vi "TimeManager.vi"(10 "Reset?":bool) -> (1 "Start Time":u32, 3 "Time Since Reset":u32)   [LabVIEW 2014]
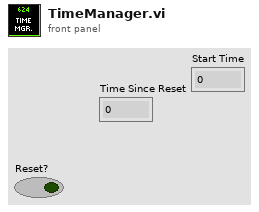
[diagram p1: front panel]
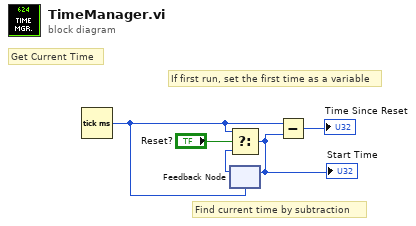
[diagram p0: block diagram]
diagram:
  # "Find current time by subtraction"
  # "If first run, set the first time as a variable"
  # "Get Current Time"
  n1 = Tick Count (ms)() -> (millisecond timer value=w2:u32)
  n2 = feedback #1(w2) -> (w4:u32)
  n3 = Select(t=w2, s="Reset?", f=w4) -> (s? t:f=w3:u32)
  "Start Time" <- w3
  n4 = feedback-in #1(w3) -> ()
  n5 = Subtract(x=w2, y=w3) -> (x-y=→"Time Since Reset":u32)
